vi "2D Commands.vi"(4 "ITX Commands in":string, 5 "maximum":dbl, 6 "X,Y,Z Labels":string[](array[string])=["current (nA)", "field (oe)", "dV/dI (Ohm)"], 7 "minimum":dbl, 8 "error in (no error)":errorcluster, 9 "Y wavename":string="yy", 10 "X wavename":string="xx", 11 "2D wavename":string="datatest.000016") -> (0 "error out":errorcluster, 3 "result string":string="Display;AppendImage 'datatest.000016'\nModifyGraph width=216,height={Aspect,1}\nLabel bottom \"current (nA)\"\nLabel left \"field (oe)\"\nModifyImage 'datatest.000016' ctab= {*,*,Rainbow,1}\n")   [LabVIEW 2019, in "LV-Data.ITX.lvclass"]
uses:
  LV-Data.ITX.lvclass
  ITX Commands/ITX Commands.lvclass
  ITX Commands/typedefs/Label--cluster.ctl
panel:
  # "Display;AppendImage '#wave2D#'\nModifyGraph width=216,height={Aspect,1}\nLabel bottom \"#labelX#\"\nLabel left \"#labelY#\"\nModifyImage '#wave2D#' ctab= {*,*,BlueHot,1}"
  # "Display;AppendImage '#wave2D#'\nModifyGraph width=216,height={Aspect,1}\nLabel bottom \"#labelX#\"\nLabel left \"#labelY#\"\nModifyImage '#wave2D#' ctab= {120,300,BlueHot,1}"
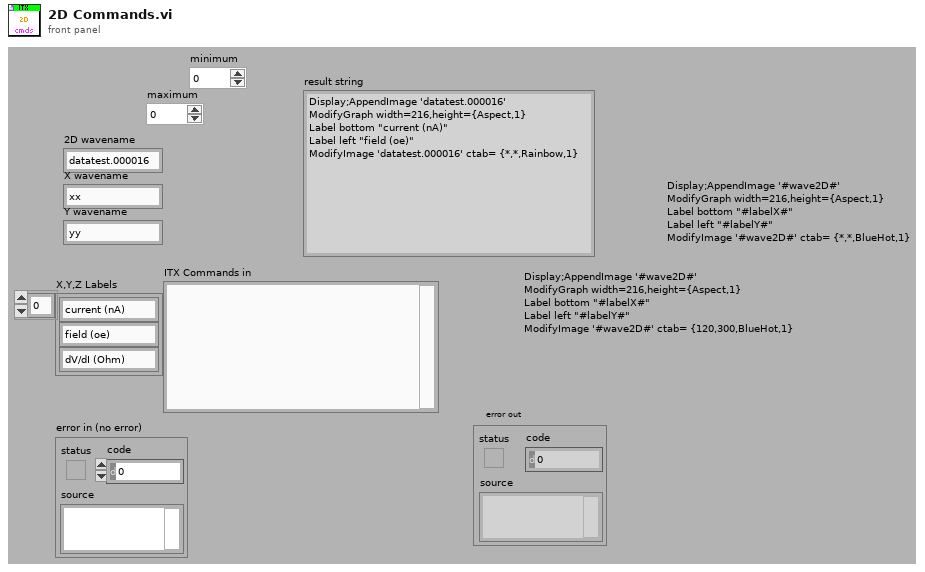
[diagram p1: front panel]
types:
  T1 = typedef "ITX Commands.lvclass/Label--cluster.ctl" = cluster{"Bottom":string, "Top":string, "Left":string, "Right":string}
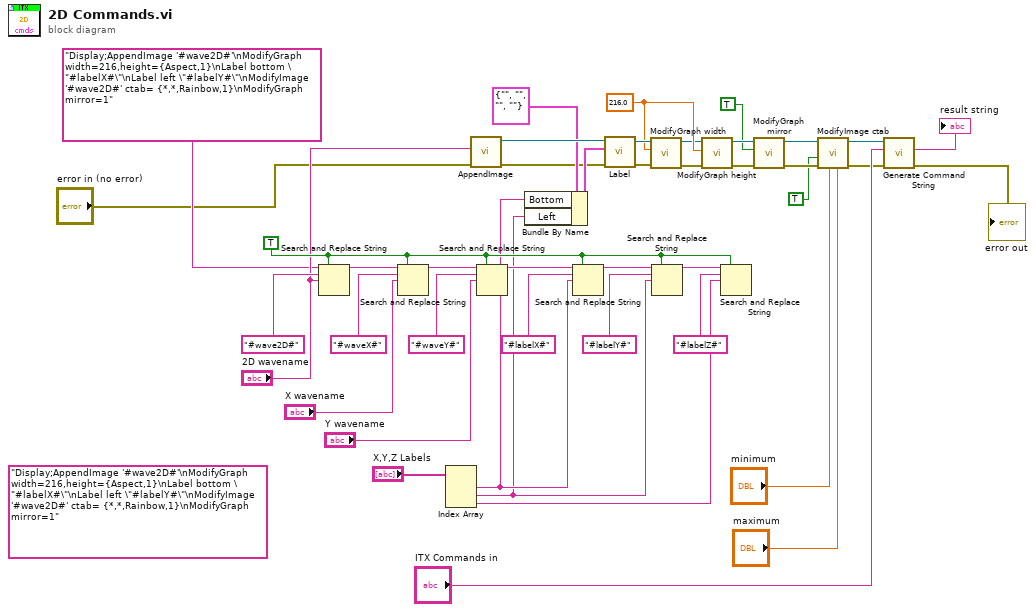
[diagram p0: block diagram]
diagram:
  (unwired) "Display;AppendImage '#wave2D#'\nModifyGraph width=216,height={Aspect,1}\nLabel bottom \"#labelX#\"\nLabel left \"#labelY#\"\nModifyImage '#wave2D#' ctab= {*,*,Rainbow,1}\nModifyGraph mirror=1" ("input command string")
  w17 = 216.0 ("width (points) [256]")
  w32 = TRUE ("replace all? (F)")
  n1 = Search and Replace String(replace all?=w32, input string="Display;AppendImage '#wave2D#'\nModifyGraph width=216,height={Aspect,1}\nLabel bottom \"#labelX#\"\nLabel left \"#labelY#\"\nModifyImage '#wave2D#' ctab= {*,*,Rainbow,1}\nModifyGraph mirror=1", search string="#wave2D#", replace string="2D wavename") -> (result string=w37:string)  [unwired: 1 in, 6 out]
  n2 = Search and Replace String(replace all?=w32, input string=w37, search string="#waveX#", replace string="X wavename") -> (result string=w39:string)  [unwired: 1 in, 6 out]
  n3 = Index Array(array="X,Y,Z Labels") -> (element #1=w23:string, element #2=w22:string, element #3=w29:string)  [unwired: 3 in]
  n4 = call "AppendImage.vi"("error in (no error)"="error in (no error)", "wavename"="2D wavename") -> ("error out"=w21:errorcluster, "ITX Commands out"=w26:refnum<class "ITX Commands.lvclass">)  [unwired: 8 in]
  n5 = Search and Replace String(replace all?=w32, input string=w39, search string="#waveY#", replace string="Y wavename") -> (result string=w33:string)  [unwired: 1 in, 6 out]
  n6 = Bundle By Name(cluster=T1 {"Bottom"="", "Top"="", "Left"="", "Right"=""} ("Label"), "Bottom"=w23, "Left"=w22) -> (w24:T1)
  n7 = Search and Replace String(replace all?=w32, input string=w33, search string="#labelX#", replace string=w23) -> (result string=w36:string)  [unwired: 1 in, 6 out]
  n8 = call "Label.vi"("error in (no error)"=w21, "Label"=w24, "ITX Commands in"=w26) -> ("error out"=w20:errorcluster, "ITX Commands out"=w19:refnum<class "ITX Commands.lvclass">)  [unwired: 7 in]
  n9 = call "ModifyGraph width.vi"("error in (no error)"=w20, "width (points) [256]"=w17, "ITX Commands in"=w19) -> ("error out"=w15:errorcluster, "ITX Commands out"=w16:refnum<class "ITX Commands.lvclass">)  [unwired: 7 in]
  n10 = Search and Replace String(replace all?=w32, input string=w36, search string="#labelY#", replace string=w22) -> (result string=w30:string)  [unwired: 1 in, 6 out]
  n11 = call "ModifyGraph height.vi"("error in (no error)"=w15, "height (points) [256]"=w17, "ITX Commands in"=w16) -> ("error out"=w13:errorcluster, "ITX Commands out"=w14:refnum<class "ITX Commands.lvclass">)  [unwired: 7 in]
  n12 = Search and Replace String(replace all?=w32, input string=w30, search string="#labelZ#", replace string=w29) -> ()  [unwired: 1 in, 7 out]
  n13 = call "ModifyGraph mirror.vi"("error in (no error)"=w13, "mirror [T]"=TRUE, "ITX Commands in"=w14) -> ("error out"=w6:errorcluster, "ITX Commands out"=w7:refnum<class "ITX Commands.lvclass">)  [unwired: 7 in]
  n14 = call "ModifyImage ctab.vi"("maximum"="maximum", "minimum"="minimum", "error in (no error)"=w6, "Invert Color Scheme? [NO]"=TRUE, "ITX Commands in"=w7) -> ("error out"=w4:errorcluster, "ITX Commands out"=w5:refnum<class "ITX Commands.lvclass">)  [unwired: 5 in]
  n15 = call "Generate Command String.vi"(0:"ITX Commands in"=w5, 1:"ITX Commands in"="ITX Commands in", "error in (no error)"=w4) -> ("ITX Commands"=→"result string":string, "error out"=→"error out":errorcluster)  [unwired: 5 in, 1 out]
